vi "Disconnect DMM.vi"(2 "error in":errorcluster, 3 "DMM Model":T1, 4 "DMM Address":refnum<visa-resource-name>="GPIB0::5::INSTR") -> (0 "error out":errorcluster)   [LabVIEW 2020]
uses:
  Typedefs/DMM Models Control.ctl
  <instrlib>/Agilent 34405/Agilent 34405.lvlib
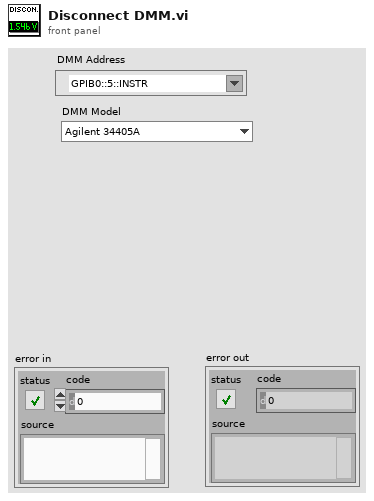
[diagram p1: front panel]
types:
  T1 = typedef "DMM Models Control.ctl" = enum16{"Agilent 34405A"}
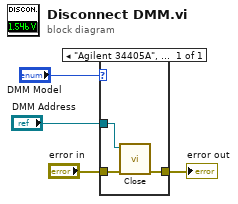
[diagram p0: block diagram]
diagram:
  n1 = case shown="\"Agilent 34405A\", Default" "DMM Model" {
    tunnel: "DMM Address" -> [w7]
    tunnel: "error in" -> [w6]
    tunnel: [w5] -> w1
    frame "Agilent 34405A", Default {
      n2 = call <instrlib>:"Close.vi"("error in (no error)"=w6, "VISA resource name"=w7) -> ("error out"=w5:errorcluster)  [unwired: 9 out]
    }
  }
  "error out" <- w1
